vi "Intake Tele-Op.vi"(9 "Buttons":bool[](array[boolean]), 10 "Axes":dbl[](array[numeric])) -> ()   [LabVIEW 2019]
uses:
  Implementation/Intake Operations.ctl
  09e80785-20b7-46c7-985e-fcded6505630.vi
  404b97f5-f42b-4c87-b346-8accad2a57ae.vi
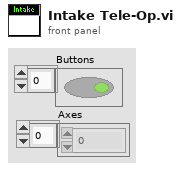
[diagram p1: front panel]
types:
  T1 = typedef "Intake Operations.ctl" = enum16{"Reserve", "Read Current", "Immediate", "Extend", "Retract"}
  T2 = cluster{"Forward Power Intake":dbl, "Operation":T1}
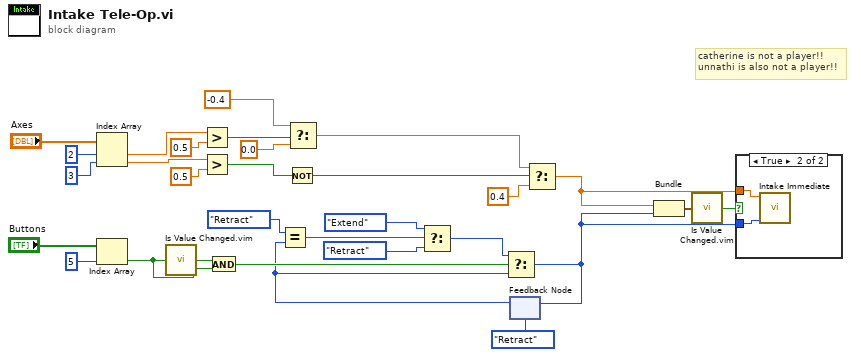
[diagram p0: block diagram]
diagram:
  # "catherine is not a player!!\nunnathi is also not a player!!"
  n1 = Index Array(array="Axes", index #1=2 ("RT"), index #2=3 ("LT")) -> (element #1=w23:dbl, element #2=w22:dbl)
  n2 = Index Array(array="Buttons", index=5 ("RB")) -> (element=w9:bool)
  n3 = call "Is Value Changed.vim"("value"=w9) -> ("changed or first call?"=w10:bool)
  n4 = Greater?(x=w23, y=0.5) -> (0:w14:bool)
  n5 = Greater?(x=w22, y=0.5) -> (0:w13:bool)
  n6 = And(x=w10, y=w9) -> (x .and. y?=w8:bool)
  n7 = Not(x=w13) -> (.not. x?=w12:bool)
  n8 = Select(t=-0.4 ("Reverse Power Intake"), s=w14, f=0.0) -> (s? t:f=w19:dbl)
  n9 = feedback #1(Intake_Operations."Retract" ("Operation")) -> (w6:T1)
  n10 = Equal?(x=Intake_Operations."Retract" ("Operation"), y=w6) -> (x = y?=w4:bool)
  n11 = Select(t=Intake_Operations."Extend" ("Operation"), s=w4, f=Intake_Operations."Retract" ("Operation")) -> (s? t:f=w1:T1)
  n12 = Select(t=w1, s=w8, f=w6) -> (s? t:f=w7:T1)
  n13 = feedback-in #1(w7) -> ()
  n14 = Select(t=w19, s=w12, f=0.4 ("Forward Power Intake")) -> (s? t:f=w17:dbl)
  n15 = Bundle("Forward Power Intake"=w17, "Operation"=w7) -> (w16:T2)  [unwired: 1 in]
  n16 = call "Is Value Changed.vim"("value"=w16) -> ("changed or first call?"=w15:bool)
  n17 = case shown="True" w15 {
    tunnel: w17 -> [_ w32]
    tunnel: w7 -> [_ w31]
    frame False {
    }
    frame True {
      n18 = call "Intake Immediate.vi"("Operation"=w31, "Intake Power"=w32) -> ()  [unwired: 10 in]
    }
  }
